vi "MonitorAlert.vi"(8 "error in (no error)":errorcluster, 10 "Str Refnum":refnum<vi>, 11 "Handle":i32) -> (0 "error out":errorcluster)   [LabVIEW 2016]
uses:
  kernel32.dll
panel:
  out "Array":u8[](array[numeric])
  out "Return":u8
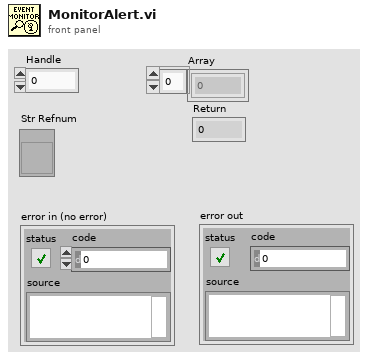
[diagram p1: front panel]
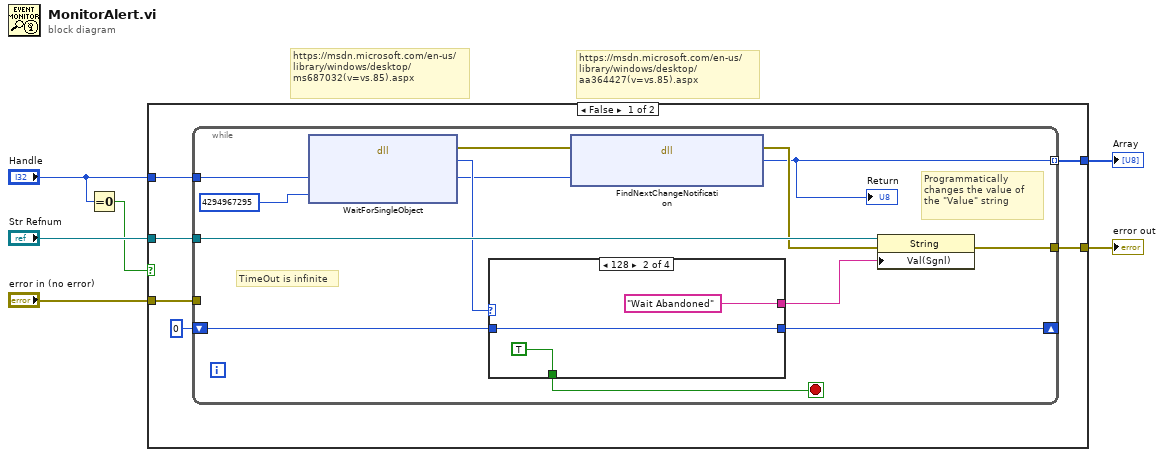
[diagram p0: block diagram]
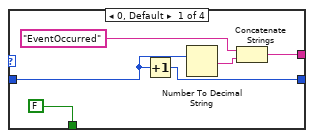
[diagram p2: hidden frame]
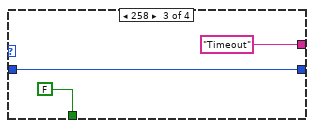
[diagram p3: hidden frame]
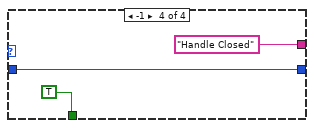
[diagram p4: hidden frame]
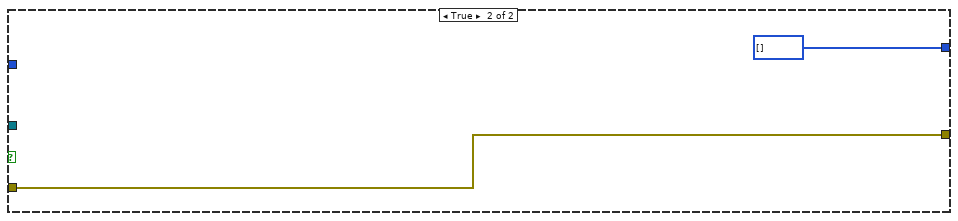
[diagram p5: hidden frame]
diagram:
  # "https://msdn.microsoft.com/en-us/library/windows/desktop/aa364427(v=vs.85).aspx"
  # "https://msdn.microsoft.com/en-us/library/windows/desktop/ms687032(v=vs.85).aspx"
  n1 = Equal To 0?(x="Handle") -> (x = 0?=w1:bool)
  n2 = case shown="False" w1 {
    tunnel: [w12 w42] -> w6
    tunnel: "Str Refnum" -> [w10 _]
    tunnel: "error in (no error)" -> [w9 w42]
    tunnel: "Handle" -> [w8 _]
    tunnel: [w7 u8[] []] -> w2
    frame False {
      n3 = while {
        tunnel: w8 -> [w22]
        tunnel: [w15] -> w12
        shift-right: [w24] -> _
        shift-left: 0 -> [w14]
        tunnel: w10 -> [w23]
        tunnel: w9 -> [_]
        tunnel: [w13] -> w7 mode=indexing
        stop <- w25 stop-if-true
        # "Programmatically changes the value of the \"Value\" string"
        # "TimeOut is infinite"
        n4 = dll-call lib="kernel32.dll" fn="WaitForSingleObject"("Handle"=w22, "dwMilliseconds"=u32 4294967295) -> (error out=w17:errorcluster, "Return"=w20:u32, "Handle"=w19:i32)  [unwired: 4 in, 1 out]
        n5 = case shown="128" w20 {
          tunnel: [w29 "Wait Abandoned" ("String") "Timeout" ("String") "Handle Closed" ("String")] -> w18
          tunnel: [FALSE TRUE FALSE TRUE] -> w25
          tunnel: w14 -> [w27 w32 w35 w38]
          tunnel: [w26 w32 w35 w38] -> w24
          frame 0, Default {
            n6 = Increment(x=w27) -> (x+1=w26:i32)
            n7 = Number To Decimal String(number=w27) -> (decimal integer string=w30:string)  [unwired: 1 in]
            n8 = Concatenate Strings("EventOccurred" ("String"), w30) -> (w29:string)
          }
          frame 128 {
          }
          frame 258 {
          }
          frame -1 {
          }
        }
        n9 = dll-call lib="kernel32.dll" fn="FindNextChangeNotification"(error in=w17, "Handle"=w19) -> (error out=w16:errorcluster, "Return"=w13:u8)  [unwired: 3 in, 1 out]
        "Return" <- w13
        n10 = property class="String"(reference=w23, error in=w16, "Val(Sgnl)"=w18) -> (error out=w15:errorcluster)  [unwired: 1 out]
      }
    }
    frame True {
    }
  }
  "error out" <- w6
  "Array" <- w2
